vi "hi_status.vi"(11 "file path":path=path "C:/luminartech/ManufacturingTools/TS_Automation/Programs/Labview/bring_up/hihb1/hihb1_resp.txt") -> (2 "Request":string, 3 "Control_mode":string)   [LabVIEW 2018]
panel:
  out "text":string
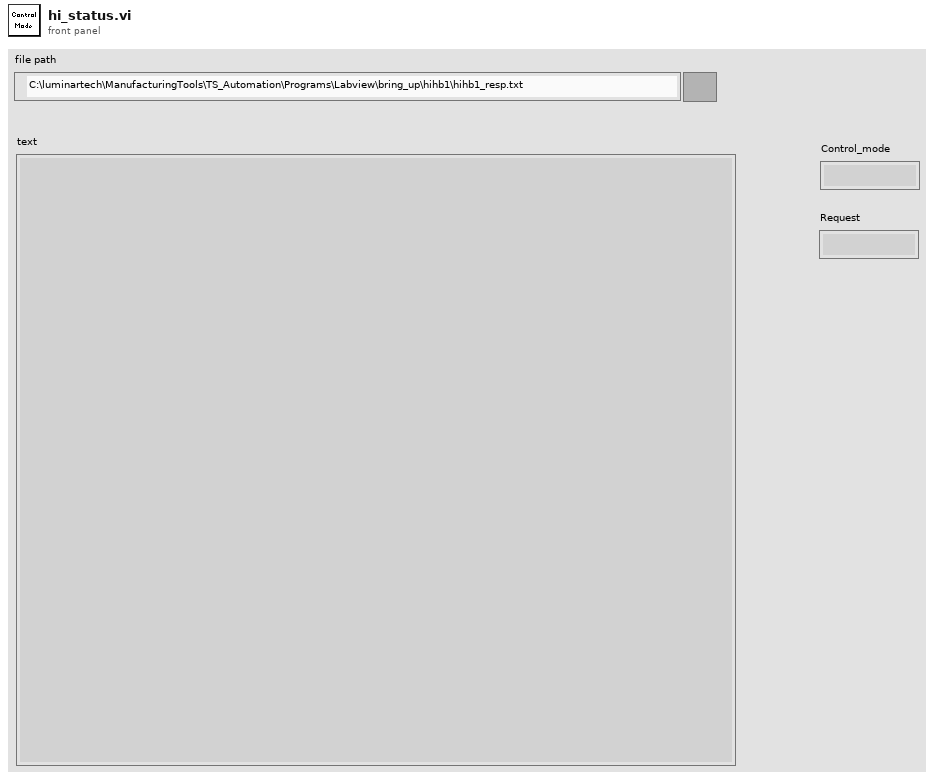
[diagram p1: front panel]
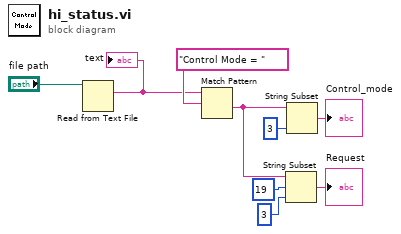
[diagram p0: block diagram]
diagram:
  n1 = Read from Text File(file (use dialog)="file path") -> (text=w5:string)  [unwired: 3 in, 3 out]
  "text" <- w5
  n2 = Match Pattern(string=w5, regular expression="Control Mode = ") -> (after substring=w2:string)  [unwired: 1 in, 3 out]
  n3 = String Subset(string=w2, offset (0)=19, length (rest)=3 ("length (rest)")) -> (substring=→"Request":string)
  n4 = String Subset(string=w2, length (rest)=3 ("length (rest)")) -> (substring=→"Control_mode":string)  [unwired: 1 in]
